vi "Log Analog Queues.vi"(8 "error in":errorcluster, 9 "Analog queues":refnum<queue>[](array[refnum]), 10 "Channel names":T1, 11 "tdms file in":refnum<k34>) -> (0 "error out":errorcluster, 3 "tdms ref out":refnum<k34>)   [LabVIEW 2020]
uses:
  <vilib>/Waveform/WDTOps.llb/WDT Get Waveform Time Array DBL.vi
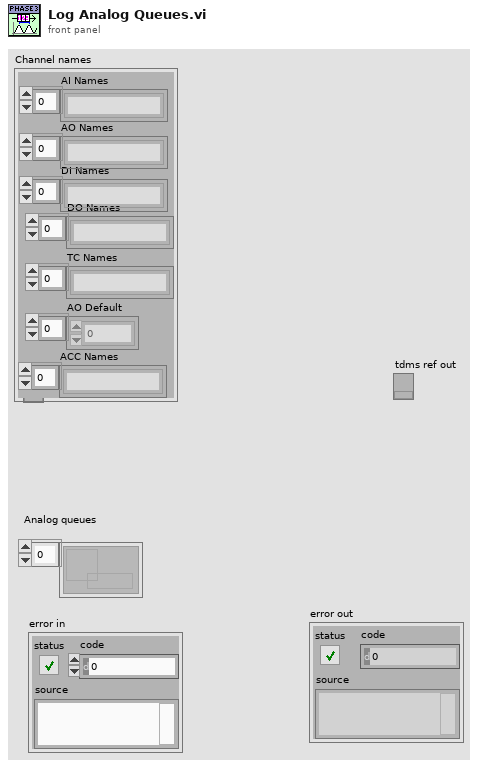
[diagram p1: front panel]
types:
  T1 = cluster{"AO Names":string[], "AI Names":string[], "DI Names":string[], "DO Names":string[], "TC Names":string[], "AO Default":dbl[], "ACC Names":string[]}
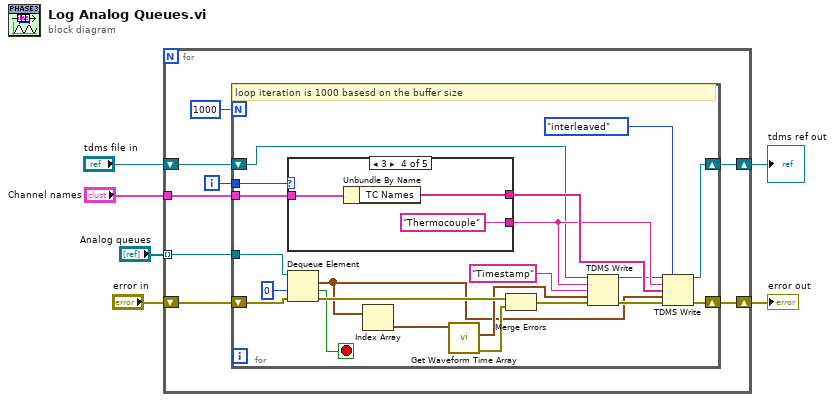
[diagram p0: block diagram]
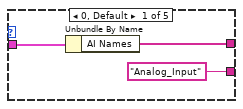
[diagram p2: hidden frame]
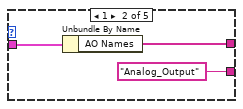
[diagram p3: hidden frame]
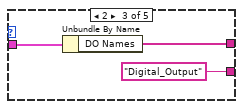
[diagram p4: hidden frame]
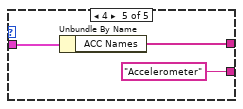
[diagram p5: hidden frame]
diagram:
  n1 = for {
    tunnel: "Analog queues" -> [w13] mode=indexing
    shift-right: [w11] -> w4
    shift-left: "tdms file in" -> [w14]
    shift-right: [w9] -> w3
    shift-left: "error in" -> [w10]
    tunnel: "Channel names" -> [w7]
    i -> [w8]
    n2 = for {
      N: 1000 -> [_]
      tunnel: w13 -> [w31]
      shift-right: [w19] -> w11
      shift-left: w14 -> [w21]
      shift-right: [w26] -> w9
      shift-left: w10 -> [w30]
      tunnel: w8 -> [w35]
      tunnel: w7 -> [w15]
      stop <- w17 stop-if-true
      # "loop iteration is 1000 basesd on the buffer size"
      n3 = case shown="3" w35 {
        tunnel: [w37 w39 w42 w45 w48] -> w25
        tunnel: ["Analog_Input" ("group name in (Untitled)") "Analog_Output" ("group name in (Untitled)") "Digital_Output" ("group name in (Untitled)") "Thermocouple" ("group name in (Untitled)") "Accelerometer" ("group name in (Untitled)")] -> w24
        tunnel: w15 -> [w36 w40 w43 w46 w49]
        frame 0, Default {
          n4 = Unbundle By Name(w36) -> ("AI Names"=w37:string[])
        }
        frame 1 {
          n5 = Unbundle By Name(w40) -> ("AO Names"=w39:string[])
        }
        frame 2 {
          n6 = Unbundle By Name(w43) -> ("DO Names"=w42:string[])
        }
        frame 3 {
          n7 = Unbundle By Name(w46) -> ("TC Names"=w45:string[])
        }
        frame 4 {
          n8 = Unbundle By Name(w49) -> ("ACC Names"=w48:string[])
        }
      }
      n9 = Dequeue Element(queue=w31, timeout in ms (-1)=0, error in (no error)=w30) -> (element=w18:waveform(dbl)[], timed out?=w17:bool, error out=w33:errorcluster)  [unwired: 1 out]
      n10 = Index Array(array=w18) -> (element=w29:waveform(dbl))  [unwired: 1 in]
      n11 = call-poly <vilib>:"Get Waveform Time Array.vi"("waveform in"=w29) -> ("error out"=w32:errorcluster, "X array"=w22:timestamp[])  [unwired: 9 in]
      n12 = Merge Errors(w33, w32) -> (w28:errorcluster)
      n13 = TDMS Write(0:w21, 5:w24, 7:"Timestamp", 9:w22, 11:w28) -> (4:w20:refnum<k34>, 15:w27:errorcluster)  [unwired: 1 in, 2 out]
      n14 = TDMS Write(0:w20, 1:enum16{"decimated", "interleaved"}."interleaved" ("data layout (0:decimated)"), 5:w24, 7:w25, 9:w18, 11:w27) -> (4:w19:refnum<k34>, 15:w26:errorcluster)  [unwired: 2 out]
    }
  }
  "tdms ref out" <- w4
  "error out" <- w3
